vi "DrivePath.vi"(2 "Parameter String":string, 3 "Reinit":bool) -> (0 "Path Follower Error":errorcluster, 1 "Increment":bool)   [LabVIEW 2020]
doc: "A pure-pursuit path-following algorithm configured for a swerve drive. Feed-forward and feed-back controllers are combined to produce unitless drive commands. This VI is designed to integrated with the FRC 4265 Autonomous Path Planner. The Search Window can be specified in seconds - longer search windows are more robust to recovering from large deviations from the path but may cause the robot to \"jump\" ahead when following tight loops or turns. The Look-Ahead Time specifies the furthest ahead the pursuit point can be.\n\nParameters:\n1. acceptable distance error --> (in) [0,614.25]\n2. acceptable angle error --> (deg) [0,180]\n3. path follow timeout --> (ms) [0,15000] set to -1 for no timeout\n3. name of the autonomous path\n4. specifiy whether or not the robot can add a suffix to the selected path name {normal,robot_suffix}"
uses:
  5c80b45a-8b82-4ca3-a7a6-7ac929992d21.vi
  SafeParser_Float.vi
  SafeParser_Integer.vi
  SafeParser_String.vi
  sensordata.vi
  autonomousinfo.vi
  drivercommands.vi
panel:
  out "PID Strafe":T1(graph)
  in  "PID Tuning Strafe":T2={"Kp"=0.03, "Ki"=0.0, "Kd"=0.0, "N-Diff"=10, "N-Int"=10, "Int Error Window"=5.0, "Max Ouput"=1.0, "Min Output"=-1.0} {"Int Error Window" min=0.0; "N-Int" min=2; "N-Diff" min=2; "Kd" min=0.0; "Ki" min=0.0; "Kp" min=0.0}
  out "PID Heading":T1(graph)
  in  "PID Tuning Heading":T2={"Kp"=0.01, "Ki"=0.0, "Kd"=0.0, "N-Diff"=10, "N-Int"=10, "Int Error Window"=30.0, "Max Ouput"=1.0, "Min Output"=-1.0} {"Int Error Window" min=0.0; "N-Int" min=2; "N-Diff" min=2; "Kd" min=0.0; "Ki" min=0.0; "Kp" min=0.0}
  out "Path and Robot Pose":cluster{dbl[], dbl[]}[](graph)
  in  "Plot":bool
  in  "Max Look-Ahead Time (s)":dbl=0.5
  in  "Search Window (s)":dbl=2.0
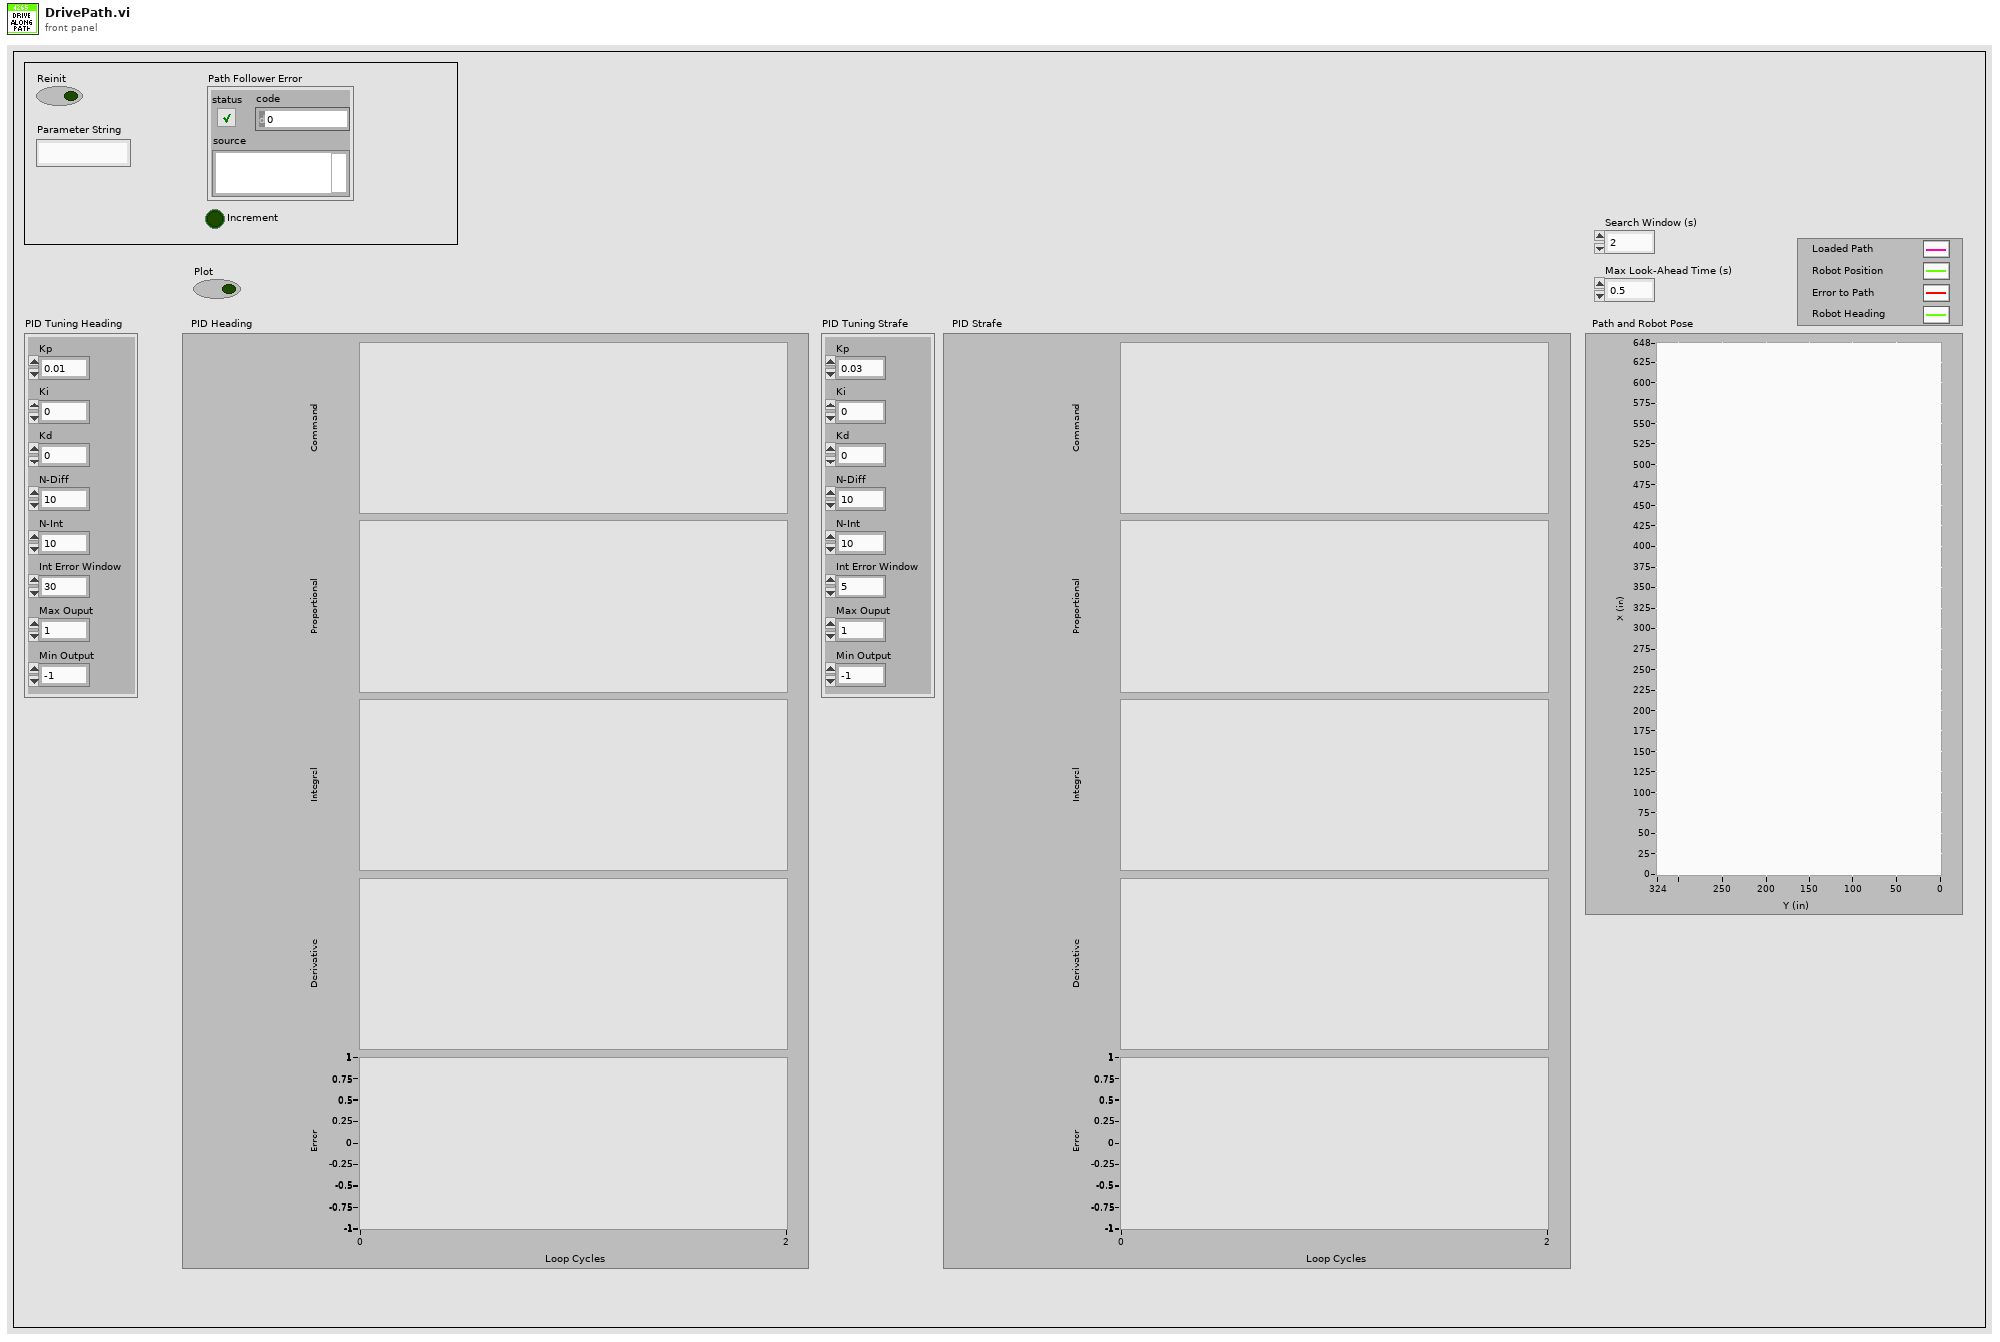
[diagram p1: front panel]
types:
  T1 = cluster{"Command":dbl, "Proportional":dbl, "Integral":dbl, "Derivative":dbl, "Goal":dbl}
  T2 = cluster{"Kp":dbl, "Ki":dbl, "Kd":dbl, "N-Diff":i32, "N-Int":i32, "Int Error Window":dbl, "Max Ouput":dbl, "Min Output":dbl}
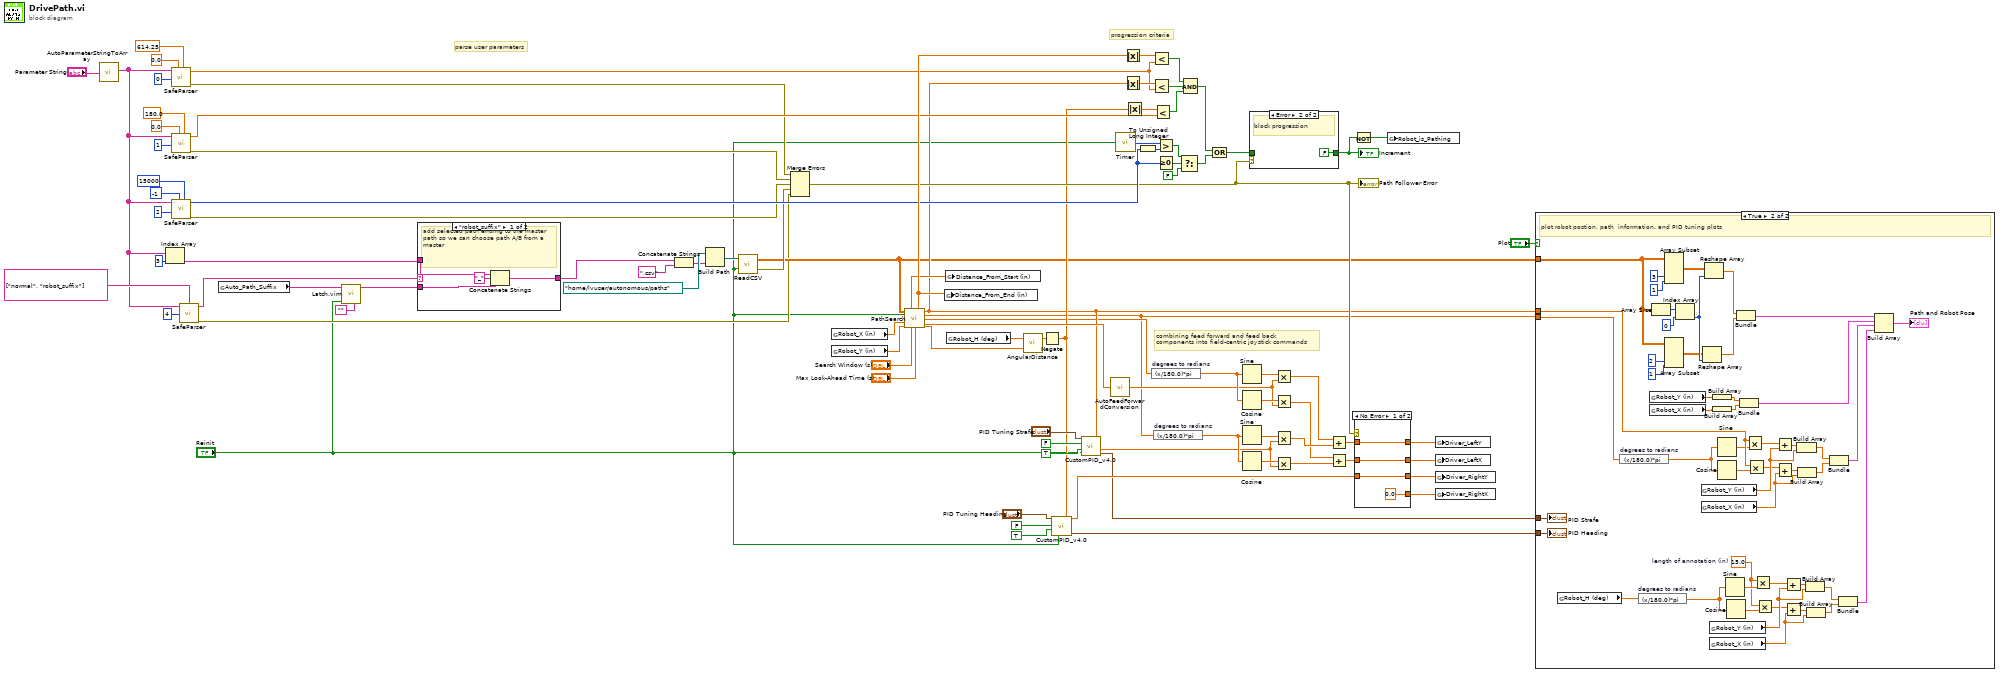
[diagram p0: block diagram]
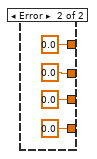
[diagram p5: hidden frame]
diagram:
  # "parse user parameters"
  # "progression criteria"
  # "combining feed forward and feed back\ncomponents into field-centric joystick commands"
  n1 = call "AutoParameterStringToArray.vi"("Parameter String"="Parameter String") -> ("Parsed Parameters"=w21:string[])
  n2 = Index Array(array=w21, index=3) -> (element=w24:string)
  n3 = call-poly "SafeParser.vi"("Maximum"=614.25, "Minimum"=0.0, "Array Index"=0 ("Parameter Index"), "String Array"=w21) -> ("Error Out"=w54:errorcluster, "Typecast  Value"=w62:dbl)  [unwired: 6 in]
  n4 = call-poly "SafeParser.vi"("Maximum"=180.0, "Minimum"=0.0, "Array Index"=1 ("Parameter Index"), "String Array"=w21) -> ("Error Out"=w55:errorcluster, "Typecast  Value"=w59:dbl)  [unwired: 6 in]
  n5 = call-poly "SafeParser.vi"("Maximum"=15000, "Minimum"=-1, "Array Index"=2 ("Parameter Index"), "String Array"=w21) -> ("Error Out"=w56:errorcluster, "Typecast  Value"=w67:i32)  [unwired: 6 in]
  n6 = call-poly "SafeParser.vi"("Allowed Values"=string[] ["normal", "robot_suffix"], "Array Index"=4, "String Array"=w21) -> ("Error Out"=w20:errorcluster, "Typecast Value"=w22:string)  [unwired: 7 in]
  n7 = global read "autonomousinfo.vi" "Auto_Path_Suffix"() -> (w6:string)
  n8 = call "Latch.vim"("Default Value"="", "Latch Signal"="Reinit", "Latch Value"=w6) -> ("Latched"=w3:string)  [unwired: 8 in]
  n9 = case shown="\"robot_suffix\"" w22 {
    tunnel: w24 -> [w97 w98]
    tunnel: [w96 w98] -> w23
    tunnel: w3 -> [w95 _]
    frame "robot_suffix" {
      # "add selected path ending to the master \npath so we can choose path A/B from a master"
      n10 = Concatenate Strings(w97, "_" ("string"), w95) -> (w96:string)
    }
    frame "normal", Default {
    }
  }
  n11 = Concatenate Strings(w23, ".csv" ("string")) -> (w87:string)
  n12 = Build Path(base path=path "/home/lvuser/autonomous/paths" ("path"), name or relative path=w87) -> (appended path=w92:path)
  n13 = call "ReadCSV.vi"("Reinit"="Reinit", "File Path (.csv)"=w92) -> ("File Open Eror"=w57:errorcluster, "Data (index by row)"=w29:dbl[][])
  n14 = Merge Errors(w54, w55, w56, w57, w20) -> (w58:errorcluster)
  "Path Follower Error" <- w58
  n15 = global read "sensordata.vi" "Robot_X (in)"() -> (w91:dbl)
  n16 = global read "sensordata.vi" "Robot_Y (in)"() -> (w90:dbl)
  n17 = call "PathSearch.vi"("Path"=w29, "Reint"="Reinit", "Robot X (in)"=w91, "Robot Y (in)"=w90, "Search Window (s)"="Search Window (s)", "Look-Ahead Time (s)"="Max Look-Ahead Time (s)") -> ("Distance from Start (in)"=w80:dbl, "Distance from End (in)"=w81:dbl, "Feed Back Distance Error (in)"=w35:dbl, "Feed Back Pointing Angle (deg)"=w14:dbl, "Feed Forward Pointing Angle (deg)"=w19:dbl, "Feed Forward Velocity (in/s)"=w82:dbl, "Robot Heading Goal (deg)"=w70:dbl)  [unwired: 3 in]
  n18 = global write "autonomousinfo.vi" "Distance_From_End (in)"(w81) -> ()
  n19 = global write "autonomousinfo.vi" "Distance_From_Start (in)"(w80) -> ()
  n20 = global read "sensordata.vi" "Robot_H (deg)"() -> (w42:dbl)
  n21 = call "AngularDistance.vi"("Goal Angle (deg) [0,360]"=w70, "Current Angle (deg) [-Inf,+Inf]"=w42) -> ("Signed Angular Distance (deg) [-180,+180]"=w40:dbl)  [unwired: 1 out]
  n22 = Negate(x=w40) -> (-x=w39:dbl)
  n23 = call "CustomPID_v4.0.vi"("PID Tuning Parameters"="PID Tuning Heading", "Custom Error Calculation"=w39, "Reset on Goal Change ?"=FALSE, "Use Custom Error Calculation ?"=TRUE, "Reinit"="Reinit") -> ("Command"=w50:dbl, "Controller Summary"=w38:T1)  [unwired: 7 in, 2 out]
  n24 = call "CustomPID_v4.0.vi"("PID Tuning Parameters"="PID Tuning Strafe", "Custom Error Calculation"=w35, "Reset on Goal Change ?"=FALSE, "Use Custom Error Calculation ?"=TRUE, "Reinit"="Reinit") -> ("Command"=w13:dbl, "Controller Summary"=w45:T1)  [unwired: 7 in, 2 out]
  n25 = call "AutoFeedForwardConversion.vi"("Target Velocity (in/s)"=w82) -> ("Equivalent Joystick Command (ul)"=w18:dbl)
  n26 = call "Timer.vi"("Reset Timer"="Reinit") -> ("Time (ms)"=w71:u32)
  n27 = Absolute Value(x=w81) -> (abs(x)=w72:dbl)
  n28 = Absolute Value(x=w35) -> (abs(x)=w73:dbl)
  n29 = Absolute Value(x=w39) -> (abs(x)=w79:dbl)
  n30 = To Unsigned Long Integer(number=w67) -> (unsigned 32bit integer=w77:u32)
  n31 = expression code="(x/180.0)*pi" "degrees to radians"(w19) -> (w85:dbl)
  n32 = Less?(x=w72, y=w62) -> (x < y?=w32:bool)
  n33 = Less?(x=w73, y=w62) -> (x < y?=w33:bool)
  n34 = Less?(x=w79, y=w59) -> (x < y?=w34:bool)
  n35 = expression code="(x/180.0)*pi" "degrees to radians"(w14) -> (w17:dbl)
  n36 = Greater?(x=w71, y=w77) -> (0:w75:bool)
  n37 = Greater Or Equal To 0?(x=w67) -> (x >= 0?=w76:bool)
  n38 = Select(t=w75, s=w76, f=FALSE) -> (s? t:f=w30:bool)
  n39 = Compound Arithmetic op=AND(w32, w33, w34) -> (w31:bool)
  n40 = Compound Arithmetic op=OR(w31, w30) -> (w78:bool)
  n41 = Sine(x=w85) -> (sin(x)=w84:dbl)
  n42 = Cosine(x=w85) -> (cos(x)=w83:dbl)
  n43 = Sine(x=w17) -> (sin(x)=w16:dbl)
  n44 = Cosine(x=w17) -> (cos(x)=w15:dbl)
  n45 = case shown="Error" w58 {
    tunnel: [w99 FALSE] -> w2
    tunnel: w78 -> [w99 _]
    frame No Error {
      # "allow progression"
    }
    frame Error {
      # "block progression"
    }
  }
  "Increment" <- w2
  n46 = Multiply(x=w84, y=w18) -> (x*y=w12:dbl)
  n47 = Multiply(x=w83, y=w18) -> (x*y=w10:dbl)
  n48 = Multiply(x=w16, y=w13) -> (x*y=w11:dbl)
  n49 = Multiply(x=w15, y=w13) -> (x*y=w9:dbl)
  n50 = Add(x=w12, y=w11) -> (x+y=w8:dbl)
  n51 = Add(x=w10, y=w9) -> (x+y=w7:dbl)
  n52 = Not(x=w2) -> (.not. x?=w1:bool)
  n53 = case shown="No Error" w58 {
    tunnel: [w101 0.0] -> w37
    tunnel: [w104 0.0 ("upper limit")] -> w86
    tunnel: [w102 0.0] -> w36
    tunnel: w50 -> [w104 _]
    tunnel: [0.0 0.0] -> w41
    tunnel: w8 -> [w102 _]
    tunnel: w7 -> [w101 _]
    frame No Error {
    }
    frame Error {
    }
  }
  n54 = global write "autonomousinfo.vi" "Robot_is_Pathing"(w1) -> ()
  n55 = global write "drivercommands.vi" "Driver_LeftY"(w36) -> ()
  n56 = global write "drivercommands.vi" "Driver_LeftX"(w37) -> ()
  n57 = global write "drivercommands.vi" "Driver_RightY"(w86) -> ()
  n58 = global write "drivercommands.vi" "Driver_RightX"(w41) -> ()
  n59 = case shown="True" "Plot" {
    tunnel: w14 -> [_ w152]
    tunnel: w45 -> [_ w151]
    tunnel: w38 -> [_ w150]
    tunnel: w35 -> [_ w149]
    tunnel: w29 -> [_ w148]
    frame False {
    }
    frame True {
      w113 = 15.0  # length of annotation (in)
      # "plot robot postion, path  information, and PID tuning plots"
      n60 = global read "sensordata.vi" "Robot_H (deg)"() -> (w153:dbl)
      n61 = expression code="(x/180.0)*pi" "degrees to radians"(w152) -> (w125:dbl)
      n62 = expression code="(x/180.0)*pi" "degrees to radians"(w153) -> (w114:dbl)
      n63 = global read "sensordata.vi" "Robot_Y (in)"() -> (w157:dbl)
      n64 = global read "sensordata.vi" "Robot_X (in)"() -> (w156:dbl)
      n65 = Array Size(array=w148) -> (size(s)=w144:i32[])
      n66 = Array Subset(array=w148, index (col)=2 ("index"), length (col)=1 ("length")) -> (w142:dbl[][])  [unwired: 2 in]
      n67 = Array Subset(array=w148, index (col)=3 ("index"), length (col)=1 ("length")) -> (w143:dbl[][])  [unwired: 2 in]
      n68 = Index Array(array=w144, index=0) -> (element=w145:i32)
      n69 = global read "sensordata.vi" "Robot_Y (in)"() -> (w135:dbl)
      n70 = global read "sensordata.vi" "Robot_X (in)"() -> (w134:dbl)
      n71 = Reshape Array(w142, w145) -> (w110:dbl[])
      n72 = Reshape Array(w143, w145) -> (w111:dbl[])
      n73 = global read "sensordata.vi" "Robot_Y (in)"() -> (w124:dbl)
      n74 = global read "sensordata.vi" "Robot_X (in)"() -> (w123:dbl)
      n75 = Build Array(w157) -> (w154:dbl[])
      n76 = Build Array(w156) -> (w155:dbl[])
      n77 = Sine(x=w125) -> (sin(x)=w126:dbl)
      n78 = Cosine(x=w125) -> (cos(x)=w127:dbl)
      n79 = Sine(x=w114) -> (sin(x)=w115:dbl)
      n80 = Cosine(x=w114) -> (cos(x)=w116:dbl)
      n81 = Bundle(w111, w110) -> (w147:cluster{dbl[], dbl[]})  [unwired: 1 in]
      n82 = Bundle(w154, w155) -> (w136:cluster{dbl[], dbl[]})  [unwired: 1 in]
      n83 = Multiply(x=w149, y=w126) -> (x*y=w128:dbl)
      n84 = Multiply(x=w149, y=w127) -> (x*y=w129:dbl)
      n85 = Multiply(x=w113, y=w115) -> (x*y=w117:dbl)
      n86 = Multiply(x=w113, y=w116) -> (x*y=w118:dbl)
      n87 = Add(x=w128, y=w135) -> (x+y=w130:dbl)
      n88 = Add(x=w129, y=w134) -> (x+y=w131:dbl)
      n89 = Add(x=w117, y=w124) -> (x+y=w119:dbl)
      n90 = Add(x=w118, y=w123) -> (x+y=w120:dbl)
      n91 = Build Array(w130, w135) -> (w132:dbl[])
      n92 = Build Array(w131, w134) -> (w133:dbl[])
      n93 = Build Array(w119, w124) -> (w121:dbl[])
      n94 = Build Array(w120, w123) -> (w122:dbl[])
      n95 = Bundle(w132, w133) -> (w112:cluster{dbl[], dbl[]})  [unwired: 1 in]
      n96 = Bundle(w121, w122) -> (w109:cluster{dbl[], dbl[]})  [unwired: 1 in]
      n97 = Build Array(w147, w136, w112, w109) -> (→"Path and Robot Pose":cluster{dbl[], dbl[]}[])
      "PID Strafe" <- w151
      "PID Heading" <- w150
    }
  }
